vi "test_CCDIsOpen.vi"() -> ()   [LabVIEW 2023]
uses:
  <vilib>/addons/_JKI Toolkits/Caraya/classes/Test/Test.lvclass
  <vilib>/addons/_JKI Toolkits/Caraya/classes/Assert/Assert.lvclass
  Source/Classes/CCD/CCD.lvclass
  Source/Classes/CCD/IsOpen.ctl
  <vilib>/addons/_JKI Toolkits/Caraya/classes/Assert/Assert Not Error.vi
  <vilib>/addons/_JKI Toolkits/Caraya/classes/Assert/Assert Equal Value and Type_Variant.vi
panel:
  out "error out":errorcluster
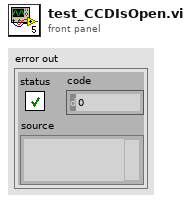
[diagram p1: front panel]
types:
  T1 = typedef "CCD.lvclass/IsOpen.ctl" = cluster{"open":bool}
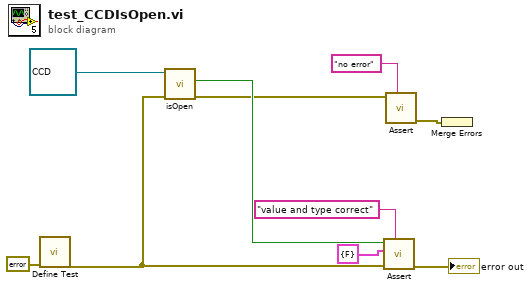
[diagram p0: block diagram]
diagram:
  n1 = call <vilib>:"Define Test.vi"("error in (no error)"=errorcluster {"status"=FALSE, "code"=0, "source"=""}) -> ("error out"=w1:errorcluster)  [unwired: 9 in, 1 out]
  n2 = call "isOpen.vi"("error in (no error)"=w1, "CCD in"=refnum<class "CCD.lvclass"> refnum) -> ("error out"=w2:errorcluster, "CCD open for communication?"=w6:bool)  [unwired: 7 in, 1 out]
  n3 = call-poly <vilib>:"Assert.vi"("Label"="value and type correct" ("Label (VI Title)"), "error in (no error)"=w1, "Y"=T1 {"open"=FALSE} ("CCD is open?"), "X"=w6) -> ("error out"=→"error out":errorcluster)  [unwired: 6 in, 1 out]
  n4 = call-poly <vilib>:"Assert.vi"("Label"="no error" ("Label (VI Title)"), "Not Error?"=w2) -> ("error out"=w3:errorcluster)  [unwired: 8 in, 1 out]
  n5 = Merge Errors(w3) -> ()  [unwired: 1 out]
